vi "simple_dac.vi"() -> ()   [LabVIEW 2017]
uses:
  lib/libbuddy/bindings/labview/utility_vi/buddy.lvlib
  <vilib>/ptbypt/NI_PtbyPt.lvlib
panel:
  out "Waveform Chart Using Bundle":cluster{u32, u32, u32, u32, u32, u32, u32, u32}(graph)
  out "Iterations":i32
  out "Time":dbl
  out "DAC Sample Time":dbl
  in  "stop":bool
  in  "frequency (Hz)":dbl=10.0 format="%0.2f"
  in  "Waveform":T1(ring)
  out "timing":cluster{"period":u32, "averaging":u8}
  in  "DAC Sample Rate (Hz)":dbl=2500.0
  out "fw_info out":T2
  out "output cluster":T3
  in  "packet":T3
  in  "timing":cluster{"period":u32, "averaging":u8}={"period"=1000000, "averaging"=0}
  in  "runtime":T4={"dac_power"=1, "dac_ref"=0, "adc_ref"=0, "adc_gain"=0}
  in  "general":T5={"function"=1, "mode"=1, "channel_mask"=255, "resolution"=1}
  out "str_serial":string
  out "str_mfr":string
  out "str_product":string
  out "str_index_1":string
  out "handle":u64 format="%x"
  # "CONFIGURATION"
  # "DEVICE INFO"
  # "DAC VALUES"
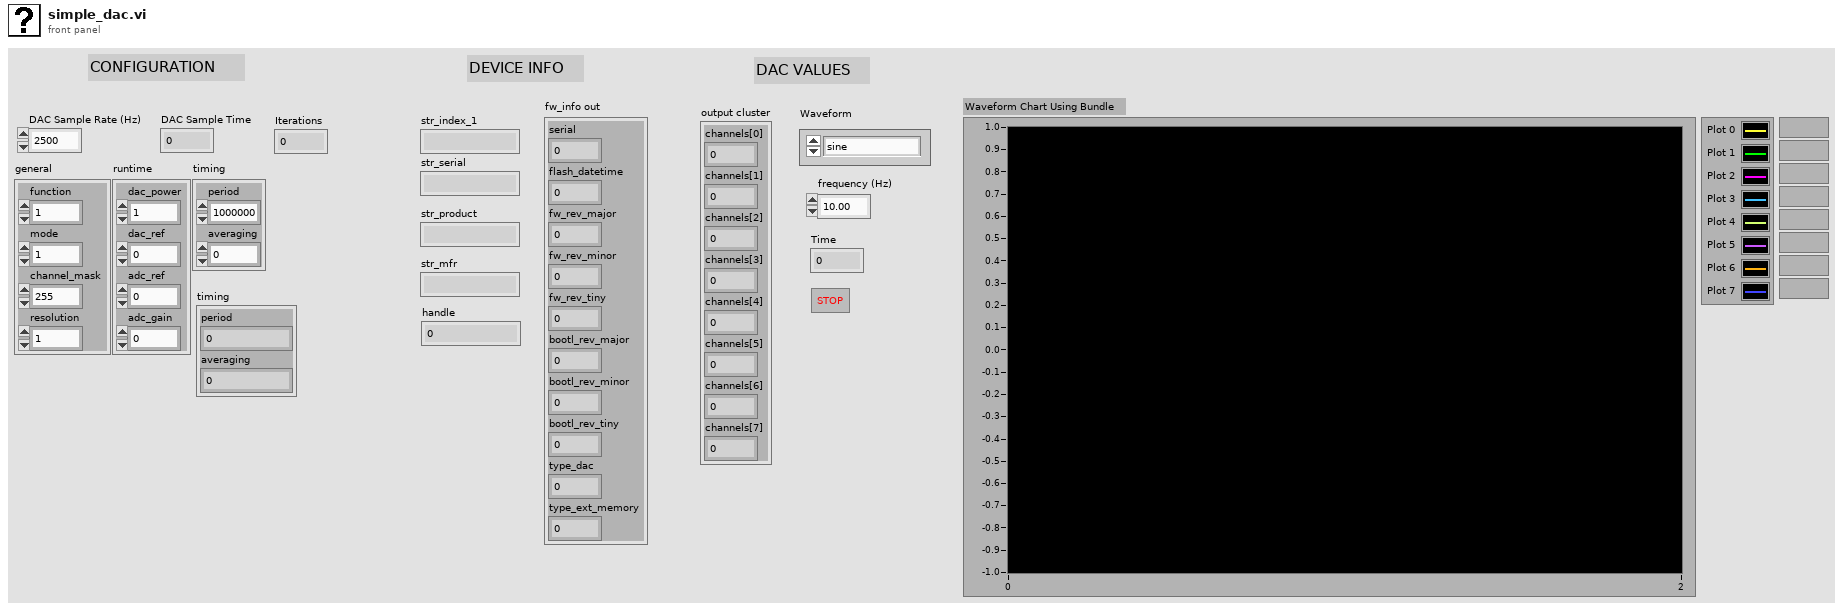
[diagram p1: front panel]
types:
  T1 = enum16{"sine", "triangle", "square", "gaussian noise"}
  T2 = cluster{"serial":u32, "flash_datetime":u32, "fw_rev_major":u8, "fw_rev_minor":u8, "fw_rev_tiny":u8, "bootl_rev_major":u8, "bootl_rev_minor":u8, "bootl_rev_tiny":u8, "type_dac":u8, "type_ext_memory":u8}
  T3 = cluster{"channels[0]":u16, "channels[1]":u16, "channels[2]":u16, "channels[3]":u16, "channels[4]":u16, "channels[5]":u16, "channels[6]":u16, "channels[7]":u16}
  T4 = cluster{"dac_power":u8, "dac_ref":u8, "adc_ref":u8, "adc_gain":u8}
  T5 = cluster{"function":u8, "mode":u8, "channel_mask":u8, "resolution":u8}
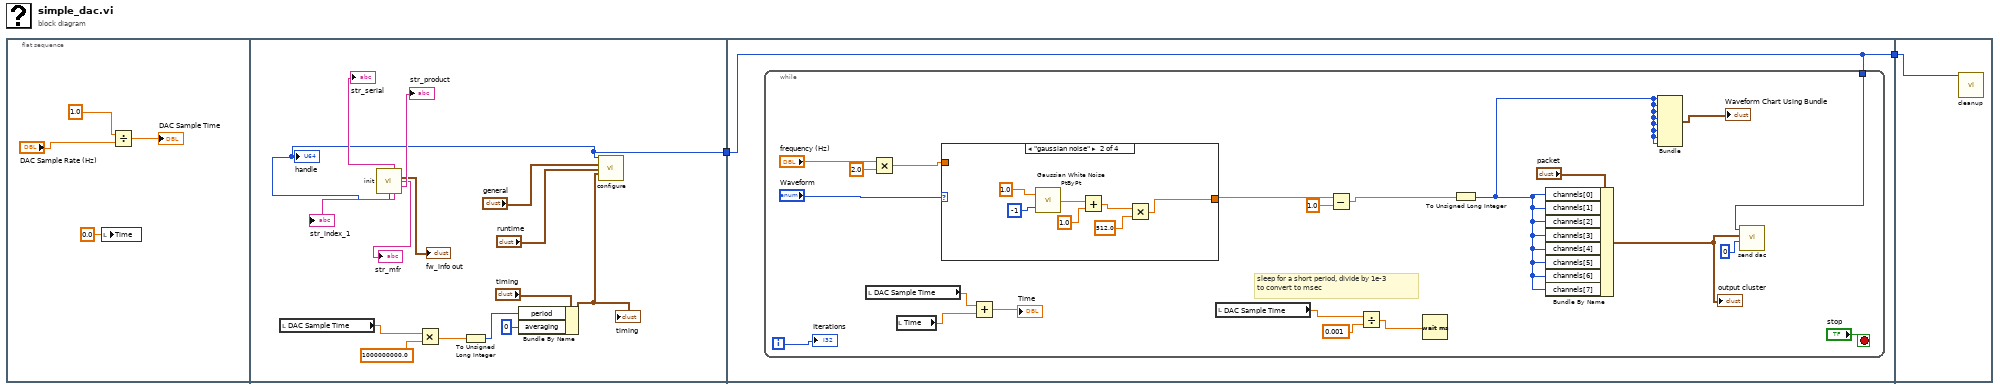
[diagram p0: block diagram]
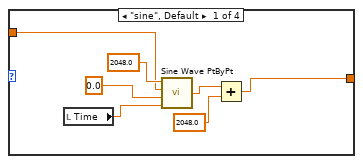
[diagram p2: hidden frame]
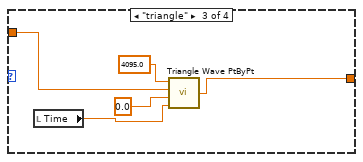
[diagram p3: hidden frame]
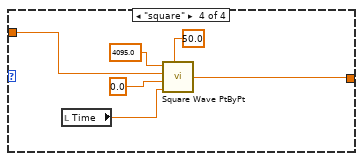
[diagram p4: hidden frame]
diagram:
  n1 = flat-sequence {
    tunnel: [w8] -> w1
    tunnel: [w22] -> w2
    tunnel: w1 -> [w22]
    tunnel: w2 -> [w69]
    frame #0 {
      n2 = local write "Time"(0.0 ("Time")) -> ()
      n3 = Divide(x=1.0, y="DAC Sample Rate (Hz)") -> (x/y=→"DAC Sample Time":dbl)
    }
    frame #1 {
      n4 = local read "DAC Sample Time"() -> (w9:dbl)
      n5 = call "init.vi"() -> ("str_serial"=→"str_serial":string, "fw_info out"=→"fw_info out":T2, "str_mfr"=→"str_mfr":string, "str_product"=→"str_product":string, "return type"=w8:u64, "str_index_1"=→"str_index_1":string)  [unwired: 8 in, 2 out]
      "handle" <- w8
      n6 = Multiply(x=w9, y=1000000000.0) -> (x*y=w12:dbl)
      n7 = To Unsigned Long Integer(number=w12) -> (unsigned 32bit integer=w11:u32)
      n8 = Bundle By Name(cluster="timing", "period"=w11, "averaging"=u8 0) -> (w14:cluster{"period":u32, "averaging":u8})
      "timing" <- w14
      n9 = call "configure.vi"("handle in"=w8, "general"="general", "runtime"="runtime", "timing"=w14) -> ()  [unwired: 7 in, 5 out]
    }
    frame #2 {
      n10 = while {
        tunnel: w22 -> [w30]
        i -> [w32]
        stop <- "stop" stop-if-true
        # "sleep for a short period, divide by 1e-3\nto convert to msec"
        n11 = local read "DAC Sample Time"() -> (w36:dbl)
        n12 = Multiply(x="frequency (Hz)", y=2.0) -> (x*y=w25:dbl)
        n13 = local read "Time"() -> (w37:dbl)
        n14 = case shown="\"gaussian noise\"" "Waveform" {
          tunnel: w25 -> [w48 _ w61 w68]
          tunnel: [w44 w51 w58 w64] -> w27
          frame "sine", Default {
            n15 = local read "Time"() -> (w47:dbl)
            n16 = call <vilib>:"Sine Wave PtByPt.vi"("time"=w47, "phase"=0.0, "frequency"=w48, "amplitude"=2048.0) -> ("sine wave"=w46:dbl)
            n17 = Add(x=w46, y=2048.0) -> (x+y=w44:dbl)
          }
          frame "gaussian noise" {
            n18 = call <vilib>:"Gaussian White Noise PtByPt.vi"("seed"=-1, "standard deviation"=1.0) -> ("Gaussian white noise"=w55:dbl)  [unwired: 1 in]
            n19 = Add(x=w55, y=1.0) -> (x+y=w53:dbl)
            n20 = Multiply(x=w53, y=512.0) -> (x*y=w51:dbl)
          }
          frame "triangle" {
            n21 = local read "Time"() -> (w59:dbl)
            n22 = call <vilib>:"Triangle Wave PtByPt.vi"("time"=w59, "phase"=0.0, "frequency"=w61, "amplitude"=4095.0) -> ("triangle wave"=w58:dbl)
          }
          frame "square" {
            n23 = local read "Time"() -> (w65:dbl)
            n24 = call <vilib>:"Square Wave PtByPt.vi"("amplitude"=4095.0, "frequency"=w68, "phase"=0.0, "time"=w65, "duty cycle (%)"=50.0) -> ("square wave"=w64:dbl)
          }
        }
        n25 = Add(x=w36, y=w37) -> (x+y=→"Time":dbl)
        n26 = local read "DAC Sample Time"() -> (w40:dbl)
        n27 = Subtract(x=w27, y=1.0) -> (x-y=w28:dbl)
        n28 = Divide(x=w40, y=0.001) -> (x/y=w41:dbl)
        n29 = Wait (ms)(milliseconds to wait=w41) -> ()  [unwired: 1 out]
        n30 = To Unsigned Long Integer(number=w28) -> (unsigned 32bit integer=w29:u32)
        n31 = Bundle By Name(cluster="packet", "channels[0]"=w29, "channels[1]"=w29, "channels[2]"=w29, "channels[3]"=w29, "channels[4]"=w29, "channels[5]"=w29, "channels[6]"=w29, "channels[7]"=w29) -> (w34:T3)
        "output cluster" <- w34
        n32 = Bundle(w29, w29, w29, w29, w29, w29, w29, w29) -> (→"Waveform Chart Using Bundle":cluster{u32, u32, u32, u32, u32, u32, u32, u32})  [unwired: 1 in]
        n33 = call "send dac.vi"("streaming"=0, "packet"=w34, "handle"=w30) -> ()  [unwired: 7 in, 2 out]
        "Iterations" <- w32
      }
    }
    frame #3 {
      n34 = call "cleanup.vi"("handle"=w69) -> ()  [unwired: 13 in, 2 out]
    }
  }
